vi "fireball Controller.vi"(8 "error in":errorcluster) -> ()   [LabVIEW 2020]
doc: "This VI executes continuously carrying out the current operation and responding to updates or new operations. It will often contain the timing or control code that is difficult to place directly in TeleOp. This VI generally opens all sensors and motors and isolates the rest of the robot code from knowing how the operations are carried out."
uses:
  <vilib>/Rock Robotics/WPI/Framework/Completion Status.ctl
  fireball Setpoints.ctl
  fireball Operations.ctl
  <vilib>/Rock Robotics/WPI/ThirdParty/Phoenix-LabVIEW/Motor Controller/Controls/CTRE_Phoenix_MotorControl_ControlMode.ctl
  <vilib>/Rock Robotics/Network Tables/NT Write Boolean.vi
panel:
  in  "Interactive Values":T1
  out "Current\nCmd":string
  in  "Buttons":cluster{"Execute Cmd":bool, "Abort Cmd":bool}
  out "Command Timing":cluster{"Start Time (ms)":u32, "Iterations":i32}
  out "Status":T3
  # "Tip: It may be helpful to observe inputs and sensor values.\nYou may also want to display tuning or debugging controls."
  # "Interactive Command: You may fill in the settings for a command\nand schedule it with the Execute button. You can observe and abort\nany command while fine tuning the code for the controller."
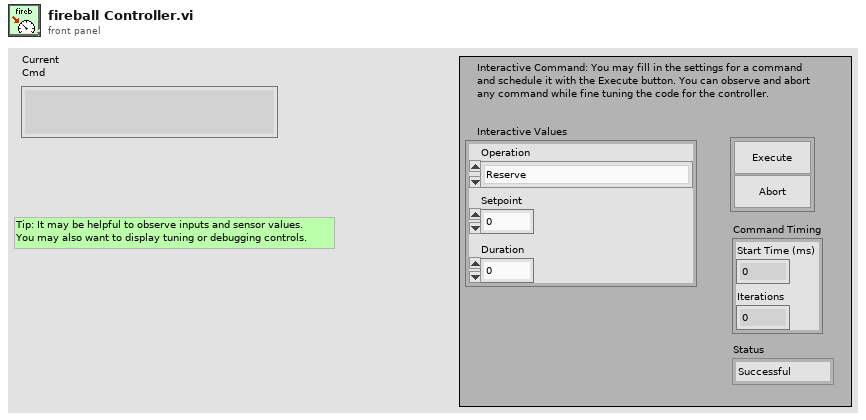
[diagram p1: front panel]
types:
  T1 = typedef "fireball Setpoints.ctl" = cluster{"Operation":T2, "Setpoint":dbl, "Duration":dbl}
  T2 = typedef "fireball Operations.ctl" = enum16{"Reserve", "Read Current", "Immediate", "fireBall"}
  T3 = typedef "Completion Status.ctl" = enum16{"Successful", "Aborted", "Incomplete"}
  T4 = typedef "WPI_MotorControlDeviceRef.ctl" = cluster{"DeviceStatus":errorcluster, "Type":T5, "PWM":cluster{"PWM Channel":T6, "DeadBand":T7}, "CAN":cluster{"Device Number":u8, "SetOutput VI Ref":variant, "GetOutput VI Ref":variant, "Enable VI Ref":variant, "Disable VI Ref":variant, "Data":variant}, "Invert":bool, "DIO PWM":cluster{"PWM \"Enable\" Channel":T6, "DIOChannel":T8, "PWM Rate":dbl}}
  T5 = typedef "WPI_MotorControlType.ctl" = enum16{"PWM", "CAN", "DIO PWM"}
  T6 = typedef "FPGA_DIOPWMChannel.ctl" = enum8{"PWM 0", "PWM 1", "PWM 2", "PWM 3", "PWM 4", "PWM 5", "PWM 6", "PWM 7", "PWM 8", "PWM 9", "PWM MXP 0", "PWM MXP 1", "PWM MXP 2", "PWM MXP 3", "PWM MXP 4", "PWM MXP 5", "PWM MXP 6", "PWM MXP 7", "PWM MXP 8", "PWM MXP 9", "Invalid"}
  T7 = typedef "WPI_PWMDeadband.ctl" = cluster{"Name":string, "maxPositivePwm":i32, "minPositivePwm":i32, "centerPwm":i32, "maxNegativePwm":i32, "minNegativePwm":i32, "angularRange":u16}
  T8 = typedef "FPGA_DIOChannel.ctl" = enum8{"DIO 0", "DIO 1", "DIO 2", "DIO 3", "DIO 4", "DIO 5", "DIO 6", "DIO 7", "DIO 8", "DIO 9", "DIO MXP 0", "DIO MXP 1", "DIO MXP 2", "DIO MXP 3", "DIO MXP 4", "DIO MXP 5", "DIO MXP 6", "DIO MXP 7", "DIO MXP 8", "DIO MXP 9", "DIO MXP 10", "DIO MXP 11", "DIO MXP 12", "DIO MXP 13", "DIO MXP 14", "DIO MXP 15", "SPI Port CS1", "SPI Port CS2", "SPI Port CS3", "SPI Port MISO", "SPI Port MOSI", "Invalid"}
  T9 = typedef "Command Status Info.ctl" = cluster{"Name":string, "Status":T3, "notifier out":T10}
  T10 = typedef "Completion Notifier.ctl" = refnum<notifier>
  T11 = cluster{"Current Command":T1, "Command Timing":cluster{"Start Time (ms)":u32, "Iterations":i32}, "Command Arguments":cluster{"Command Info":T9, "Description":string, "Default Command":T1, "queue out":refnum<queue>, "Subsystem Name":string}}
  T12 = typedef "CTRE_Phoenix_MotorControl_ControlMode.ctl" = u16
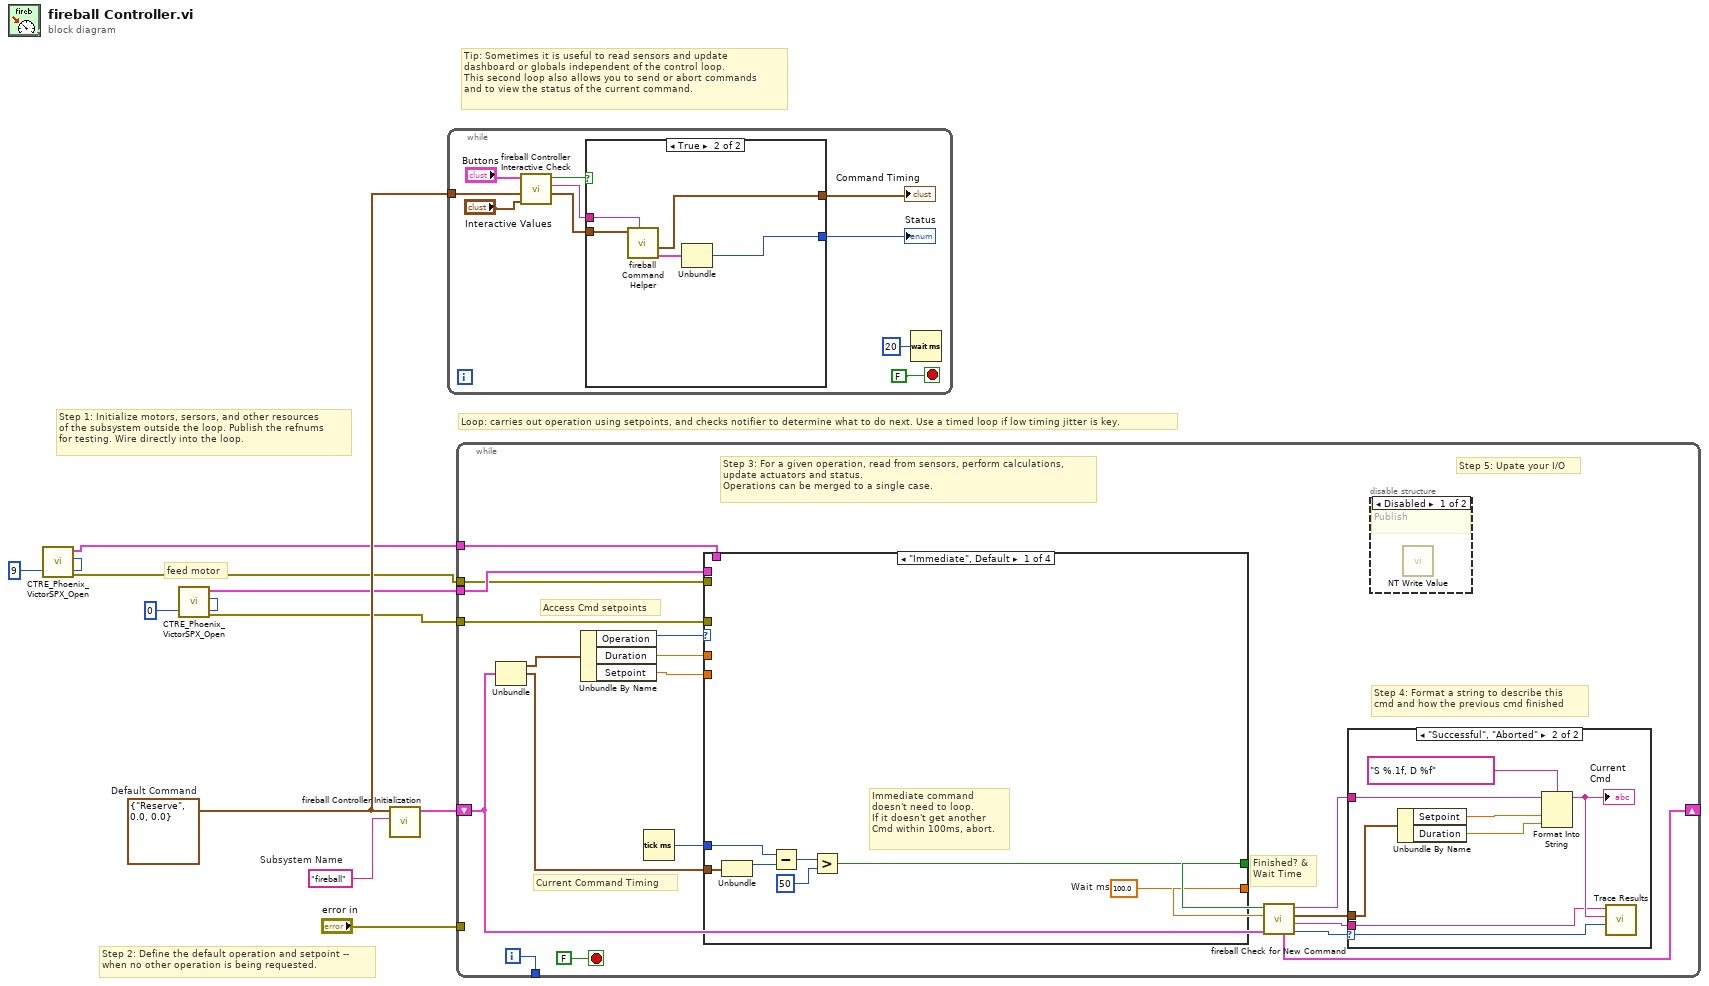
[diagram p0: block diagram]
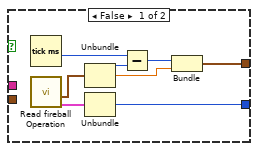
[diagram p2: hidden frame]
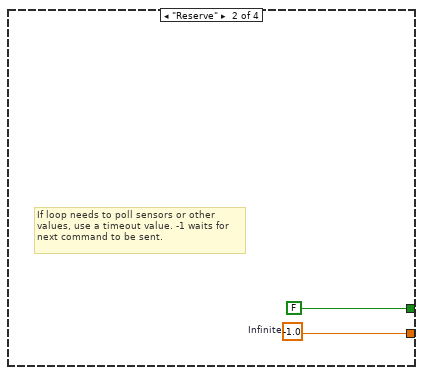
[diagram p5: hidden frame]
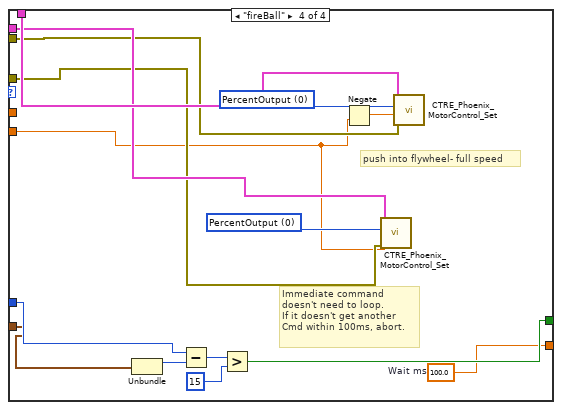
[diagram p7: hidden frame]
diagram:
  w7 = T1 {"Operation"=enum."Reserve", "Setpoint"=0.0, "Duration"=0.0}  # Default Command
  w8 = "fireball"  # Subsystem Name
  # "feed motor"
  # "Tip: Sometimes it is useful to read sensors and update\ndashboard or globals independent of the control loop.\nThis second loop also allows you to send or abort commands\nand to view the status of the current command."
  # "Step 2: Define the default operation and setpoint --\nwhen no other operation is being requested."
  # "Step 1: Initialize motors, sersors, and other resources\nof the subsystem outside the loop. Publish the refnums\nfor testing. Wire directly into the loop."
  # "Loop: carries out operation using setpoints, and checks notifier to determine what to do next. Use a timed loop if low timing jitter is key."
  n1 = call <vilib>:"CTRE_Phoenix_VictorSPX_Open.vi"("Device Number"=u8 9) -> ("error out"=w2:errorcluster, "PhoenixMotorControlDevRef"=w4:T4)  [unwired: 9 in]
  n2 = call <vilib>:"CTRE_Phoenix_VictorSPX_Open.vi"("Device Number"=u8 0) -> ("error out"=w1:errorcluster, "PhoenixMotorControlDevRef"=w3:T4)  [unwired: 9 in]
  n3 = call "fireball Controller Initialization.vi"("Subsystem Name"=w8, "Default Command"=w7) -> ("Current Command"=w9:T11)  [unwired: 9 in]
  n4 = while {
    tunnel: w7 -> [w17]
    stop <- FALSE stop-if-true
    n5 = call "fireball Controller Interactive Check.vi"("Interactive Command in"="Interactive Values", "Default Command"=w17, "Buttons"="Buttons") -> ("Interactive Command out"=w14:T1, "Trace String"=w15:string, "Schedule"=w16:bool)  [unwired: 6 in]
    n6 = case shown="True" w16 {
      tunnel: [w28 w33] -> w13
      tunnel: w14 -> [_ w31]
      tunnel: [w24 w29] -> w12
      tunnel: w15 -> [_ w32]
      frame False {
        n7 = Tick Count (ms)() -> (millisecond timer value=w23:u32)
        n8 = call "Read fireball Operation.vi"() -> ("Command Info"=w21:T9, "SubSystem Data"=w22:T1)  [unwired: 9 in, 1 out]
        n9 = Unbundle(w22) -> ("Operation"=w27:T2, "Setpoint"=w25:dbl)  [unwired: 1 out]
        n10 = Unbundle(w21) -> ("Status"=w28:T3)  [unwired: 2 out]
        n11 = Subtract(x=w23, y=w27) -> (x-y=w26:u32)
        n12 = Bundle(w26, "Setpoint"=w25) -> (w24:cluster{u32, "Setpoint":dbl})  [unwired: 1 in]
      }
      frame True {
        n13 = call "fireball Command Helper.vi"("Description"=w32, "SubSystem Data"=w31) -> ("Command Info Out"=w30:T9, "Command Timing"=w29:cluster{"Start Time (ms)":u32, "Iterations":i32})  [unwired: 7 in, 1 out]
        n14 = Unbundle(w30) -> ("Status"=w33:T3)  [unwired: 2 out]
      }
    }
    "Status" <- w13
    "Command Timing" <- w12
    n15 = Wait (ms)(milliseconds to wait=u32 20) -> ()  [unwired: 1 out]
  }
  n16 = while {
    shift-right: [w45] -> _
    shift-left: w9 -> [w38]
    tunnel: [w52] -> _
    tunnel: "error in" -> [_]
    tunnel: w4 -> [w37]
    tunnel: w3 -> [w36]
    tunnel: w2 -> [w35]
    tunnel: w1 -> [w34]
    i -> [w52]
    stop <- FALSE stop-if-true
    # "Step 5: Upate your I/O"
    # "Step 4: Format a string to describe this\ncmd and how the previous cmd finished"
    # "Current Command Timing"
    # "Access Cmd setpoints"
    # "Finished? &\nWait Time"
    # "Step 3: For a given operation, read from sensors, perform calculations,\nupdate actuators and status.\nOperations can be merged to a single case."
    n17 = Unbundle(w38) -> ("Current Command"=w51:T1, "Command Timing"=w47:cluster{"Start Time (ms)":u32, "Iterations":i32})  [unwired: 1 out]
    n18 = Unbundle By Name(w51) -> ("Operation"=w50:T2, "Duration"=w49:dbl, "Setpoint"=w46:dbl)
    n19 = Tick Count (ms)() -> (millisecond timer value=w48:u32)
    n20 = case shown="\"Immediate\", Default" w50 {
      tunnel: [w68 w70 _ w76] -> w43
      tunnel: [w62 FALSE ("ignore previous (F)") _ w77] -> w44
      tunnel: w47 -> [w64 _ _ w78]
      tunnel: w49 -> [_ _ _ _]
      tunnel: w48 -> [w63 _ _ w79]
      tunnel: w46 -> [_ _ _ w71]
      tunnel: w37 -> [_ _ _ w75]
      tunnel: w36 -> [_ _ _ w74]
      tunnel: w35 -> [_ _ _ w73]
      tunnel: w34 -> [_ _ _ w72]
      frame "Immediate", Default {
        w68 = 100.0  # Wait ms
        # "Immediate command\ndoesn't need to loop.\nIf it doesn't get another\nCmd within 100ms, abort."
        n21 = Unbundle(w64) -> ("Start Time (ms)"=w67:u32)  [unwired: 1 out]
        n22 = Subtract(x=w63, y=w67) -> (x-y=w66:u32)
        n23 = Greater?(x=w66, y=u8 50 ("Left Motor")) -> (0:w62:bool)
      }
      frame "Reserve" {
        w70 = -1.0  # Infinite
        # "If loop needs to poll sensors or other\nvalues, use a timeout value. -1 waits for\nnext command to be sent."
      }
      frame "Read Current" {
      }
      frame "fireBall" {
        w76 = 100.0  # Wait ms
        w84 = T12 0 items=["PercentOutput"=0, "Position"=1, "Velocity"=2, "Current"=3, "Follower"=5, "MotionProfile"=6, "MotionMagic"=7, "MotionProfileArc"=10, "Disabled"=15] ("Control Mode")
        w85 = T12 0 items=["PercentOutput"=0, "Position"=1, "Velocity"=2, "Current"=3, "Follower"=5, "MotionProfile"=6, "MotionMagic"=7, "MotionProfileArc"=10, "Disabled"=15] ("Control Mode")
        # "Immediate command\ndoesn't need to loop.\nIf it doesn't get another\nCmd within 100ms, abort."
        # "push into flywheel- full speed"
        n24 = Unbundle(w78) -> ("Start Time (ms)"=w81:u32)  [unwired: 1 out]
        n25 = Subtract(x=w79, y=w81) -> (x-y=w82:u32)
        n26 = Greater?(x=w82, y=u8 15 ("Left Motor")) -> (0:w77:bool)
        n27 = Negate(x=w71) -> (-x=w83:dbl)
        n28 = call <vilib>:"CTRE_Phoenix_MotorControl_Set.vi"("error in (no error)"=w72, "Output"=w71, "Control Mode"=w84, "PhoenixMotorControlDevRef"=w74) -> ()  [unwired: 6 in, 2 out]
        n29 = call <vilib>:"CTRE_Phoenix_MotorControl_Set.vi"("error in (no error)"=w73, "Output"=w83, "Control Mode"=w85, "PhoenixMotorControlDevRef"=w75) -> ()  [unwired: 6 in, 2 out]
      }
    }
    n30 = call "fireball Check for New Command.vi"("Current Command"=w38, "Wait time (ms)"=w43, "Finished?"=w44) -> ("Completion"=w39:T3, "Subsystem Name"=w40:string, "Current Command"=w41:T1, "Initial Trace String"=w42:string, "NextCommand"=w45:T11)  [unwired: 4 in]
    n31 = case shown="\"Successful\", \"Aborted\"" w39 {
      selector: w39 -> [_ w61]
      tunnel: w42 -> [_ w57]
      tunnel: w41 -> [_ w58]
      tunnel: w40 -> [_ w54]
      frame "Incomplete", Default {
        # "Continuing current command"
      }
      frame "Successful", "Aborted" {
        # "Report and setup for next command"
        n32 = Unbundle By Name(w58) -> ("Setpoint"=w60:dbl, "Duration"=w55:dbl)
        n33 = Format Into String(format string="S %.1f, D %f", initial string=w57, w60, w55) -> (resulting string=w56:string)  [unwired: 1 in, 1 out]
        "Current\nCmd" <- w56
        n34 = call <vilib>:"Trace Results.vi"("Status of previous command"=w61, "Description"=w56, "Subsystem"=w54) -> ()  [unwired: 9 in]
      }
    }
    n35 = disable-structure shown="Disabled" {
      frame Disabled {
        # "Publish"
        n36 = call-poly <vilib>:"NT Write Value.vi"() -> ()  [unwired: 11 in, 1 out]
      }
      frame Enabled {
      }
    }
  }
